vi "Maltsev fuction.vi"(1 "Angles":sgl[](array[numeric])=[1.7463206, 1.8518518, 1.365077, 82.16]) -> (0 "Maltsev fuction":dbl[](array[numeric]))   [LabVIEW 2018]
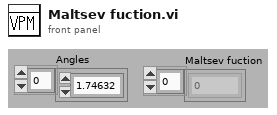
[diagram p1: front panel]
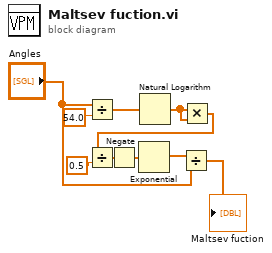
[diagram p0: block diagram]
diagram:
  n1 = Divide(x="Angles", y=54.0 ("x")) -> (x/y=w9:dbl[])
  n2 = Natural Logarithm(1:w9) -> (0:w8:dbl[])
  n3 = Multiply(x=w8, y=w8) -> (x*y=w2:dbl[])
  n4 = Divide(x=w2, y=0.5 ("x")) -> (x/y=w6:dbl[])
  n5 = Negate(x=w6) -> (-x=w4:dbl[])
  n6 = Exponential(1:w4) -> (0:w5:dbl[])
  n7 = Divide(x=w5, y="Angles") -> (x/y=→"Maltsev fuction":dbl[])
